vi "SSH OpenSSH SFTP FGV.vi"(8 "error in (no error)":errorcluster, 9 "OpenSSH Session Op":T1, 10 "OpenSSH Session in":refnum<class "Session.lvclass">, 11 "OpenSSH SFTP in":refnum<class "OpenSSH Client.lvclass">) -> (0 "error out":errorcluster, 2 "OpenSSH Session out":refnum<class "Session.lvclass">, 3 "OpenSSH SFTP out":refnum<class "OpenSSH Client.lvclass">)   [LabVIEW 2024, in "LMH-LINX.lvlib"]
uses:
  <vilib>/MakerHub/LINX/LMH-LINX.lvlib
  <vilib>/net/SSH/Client/OpenSSH/OpenSSH Client.lvclass
  <vilib>/MakerHub/LINX/Private/Utilties/SSH/SSH OpenSSH Session Op.ctl
  <vilib>/net/SFTP/Session/Session.lvclass
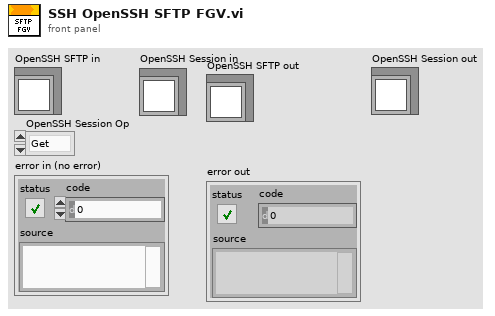
[diagram p1: front panel]
types:
  T1 = typedef "LMH-LINX.lvlib/SSH OpenSSH Session Op.ctl" = enum16{"Get", "Set"}
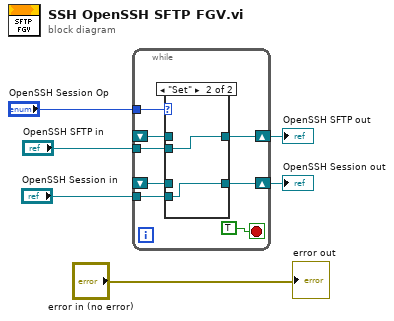
[diagram p0: block diagram]
diagram:
  n1 = while {
    shift-right: [w11] -> w4
    shift-left: _ -> [w10]
    tunnel: "OpenSSH Session Op" -> [w13]
    tunnel: "OpenSSH SFTP in" -> [w12]
    tunnel: "OpenSSH Session in" -> [w9]
    shift-right: [w8] -> w1
    shift-left: _ -> [w7]
    stop <- TRUE stop-if-true
    n2 = case shown="\"Set\"" w13 {
      tunnel: w12 -> [_ w18]
      tunnel: [w16 w18] -> w11
      tunnel: w10 -> [w16 _]
      tunnel: w9 -> [_ w17]
      tunnel: [w15 w17] -> w8
      tunnel: w7 -> [w15 _]
      frame "Get", Default {
      }
      frame "Set" {
      }
    }
  }
  "OpenSSH SFTP out" <- w4
  "OpenSSH Session out" <- w1
  "error out" <- "error in (no error)"
